vi "PV Digiline Pressure Set Point.vi"(8 "error in (no error)":errorcluster, 9 "HV                  <->                  Atm.":bool=TRUE, 10 "Adress of unit":u16=1 max=999 step=1, 11 "VISA session":refnum<visa-resource-name>) -> (0 "error out":errorcluster, 3 "dup VISA session":refnum<visa-resource-name>)   [LabVIEW 2012, in "Pfeiffer Vacuum.lvlib"]
doc: "VI for egualizing the Transmitter.\n \nTo equalize a transmitter there must first be set a pressure adjustment point (set parameter 741\n(pressure set point) to \"000 (HV)\" for low pressure or to \"001 (Atm.)\" for high pressure), and than the actual pressure value (parameter 740 (Digiline Data.VI) to the actual pressure, for example \"1000\" for 1000 mbar). \n\nWarning :\nIf the setting for the pressure adjustment point is missing or if another telegram is inserted between the two steps, an error signal is generated when writing the pressure value."
uses:
  <instrlib>/Pfeiffer Vacuum/Pfeiffer Vacuum.lvlib
panel:
  # "Pressure set point  Atm. / HV      :"
  # "<-------------\n HV"
  # "------------->          \nAtm."
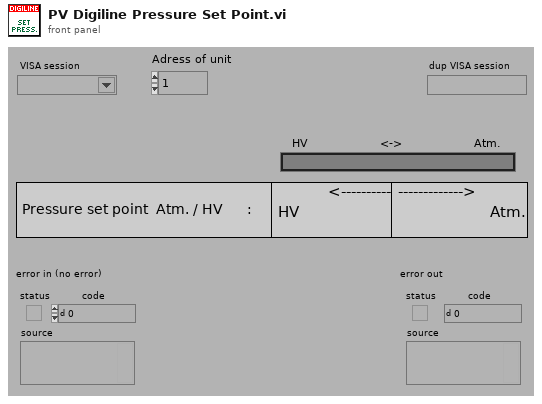
[diagram p1: front panel]
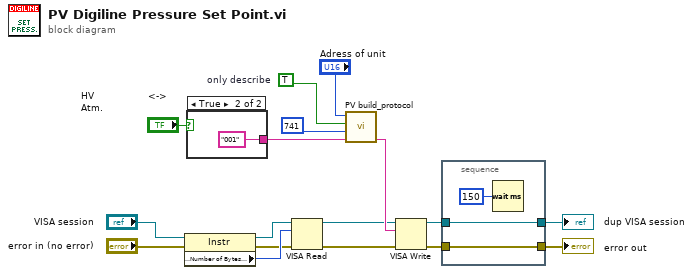
[diagram p0: block diagram]
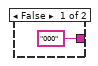
[diagram p2: hidden frame]
diagram:
  w3 = TRUE  # only describe
  n1 = property class="Instr"(reference="VISA session", error in="error in (no error)") -> (reference out=w12:refnum<visa-resource-name>, error out=w11:errorcluster, "Serial Settings:Number of Bytes at Serial Port"=w13:u32)
  n2 = case shown="TRUE" "HV                  <->                  Atm." {
    tunnel: ["000" ("Data") "001" ("Data")] -> w4
    frame False {
    }
    frame True {
    }
  }
  n3 = VISA Read(VISA resource name=w12, byte count=w13, error in (no error)=w11) -> (VISA resource name out=w10:refnum<visa-resource-name>, error out=w7:errorcluster)  [unwired: 2 out]
  n4 = call <instrlib>:"PV build_protocol.vi"("Data"=w4, "Parameter-number"=u16 741, "parameter\nread<->describe"=w3, "Adress"="Adress of unit") -> ("output"=w14:string)  [unwired: 3 in]
  n5 = VISA Write(VISA resource name=w10, write buffer=w14, error in (no error)=w7) -> (VISA resource name out=w16:refnum<visa-resource-name>, error out=w15:errorcluster)  [unwired: 1 out]
  n6 = stacked-sequence {
    tunnel: w16 -> [w22]
    tunnel: w15 -> [w21]
    tunnel: [w22] -> w2
    tunnel: [w21] -> w1
    frame #0 {
      n7 = Wait (ms)(milliseconds to wait=u32 150 ("ms Wartezeit")) -> ()  [unwired: 1 out]
    }
  }
  "error out" <- w1
  "dup VISA session" <- w2
